vi "Best fit axis-aligned ellipse.vi"(0 "x array":dbl[](array[numeric]), 1 "y array":dbl[](array[numeric])) -> (2 "x centre":dbl, 3 "y centre":dbl, 4 "x radius":dbl, 5 "y radius":dbl)   [LabVIEW 2014]
doc: "Finds the best fit axis-aligned ellipse using a non-linear least squares method. Input arrays (corresponding values of x and y) must have a minimum of 4 values each"
uses:
  <vilib>/Analysis/baseanly.llb/Real A x B.vi
  <vilib>/Analysis/baseanly.llb/A x Vector.vi
  <vilib>/Analysis/Matrix/Numeric/Conversions/Array To Matrix - RA2.vi
  <vilib>/Analysis/baseanly.llb/Real Inverse Matrix.vi
  <vilib>/Analysis/Matrix/NI_Matrix.lvlib
  <vilib>/Analysis/NI_AALBase.lvlib
panel:
  # "Paul Nathan 24/06/2015"
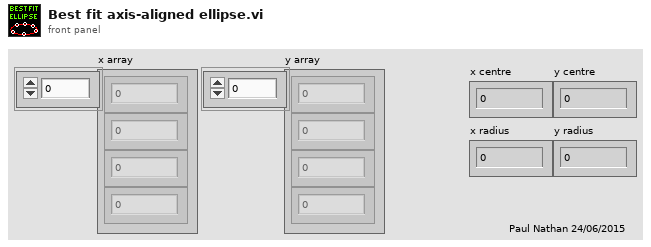
[diagram p1: front panel]
types:
  T1 = typedef "NI_Matrix.lvlib/RealMatrix.ctl" = dbl[][]
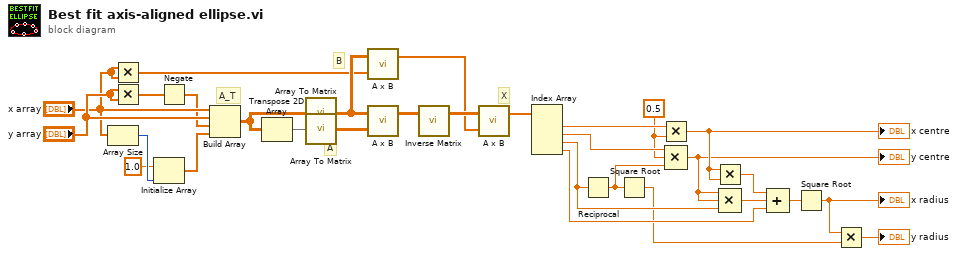
[diagram p0: block diagram]
diagram:
  w16 = 0.5 ("y")
  # "A_T"
  # "X"
  # "A"
  # "B"
  n1 = Array Size(array="x array") -> (size(s)=w30:i32)
  n2 = Multiply(x="x array", y="x array") -> (x*y=w10:dbl[])
  n3 = Multiply(x="y array", y="y array") -> (x*y=w9:dbl[])
  n4 = Initialize Array(1.0 ("element"), w30) -> (w11:dbl[])
  n5 = Negate(x=w9) -> (-x=w8:dbl[])
  n6 = Build Array("x array", "y array", w8, w11) -> (w25:dbl[][])
  n7 = Transpose 2D Array(2D array=w25) -> (transposed array=w26:dbl[][])
  n8 = call-poly <vilib>:"Array To Matrix.vi"("Real 2D Array"=w25) -> ("Real Matrix"=w23:T1)
  n9 = call-poly <vilib>:"Array To Matrix.vi"("Real 2D Array"=w26) -> ("Real Matrix"=w24:T1)
  n10 = call-poly <vilib>:"A x B.vi"("Vector"=w10, "A"=w23) -> ("A x Vector"=w20:dbl[])  [unwired: 1 out]
  n11 = call-poly <vilib>:"A x B.vi"("B"=w24, "A"=w23) -> ("A x B"=w22:T1)  [unwired: 1 out]
  n12 = call-poly <vilib>:"Inverse Matrix.vi"("Input Matrix"=w22) -> ("Inverse Matrix"=w21:T1)  [unwired: 1 in, 1 out]
  n13 = call-poly <vilib>:"A x B.vi"("Vector"=w20, "A"=w21) -> ("A x Vector"=w19:dbl[])  [unwired: 1 out]
  n14 = Index Array(array=w19) -> (element #1=w18:dbl, element #2=w17:dbl, element #3=w5:dbl, element #4=w7:dbl)  [unwired: 4 in]
  n15 = Reciprocal(x=w5) -> (1/x=w6:dbl)
  n16 = Square Root(x=w6) -> (sqrt(x)=w2:dbl)
  n17 = Multiply(x=w18, y=w16) -> (x*y=w15:dbl)
  "x centre" <- w15
  n18 = Compound Arithmetic op=MULTIPLY(w17, w16, w6) -> (w14:dbl)
  "y centre" <- w14
  n19 = Multiply(x=w15, y=w15) -> (x*y=w13:dbl)
  n20 = Compound Arithmetic op=MULTIPLY(w14, w14, w5) -> (w4:dbl)
  n21 = Compound Arithmetic op=ADD(w13, w4, w7) -> (w12:dbl)
  n22 = Square Root(x=w12) -> (sqrt(x)=w3:dbl)
  "x radius" <- w3
  n23 = Multiply(x=w3, y=w2) -> (x*y=→"y radius":dbl)
